vi "Close FPGA Ref.vi"(8 "error in (no error)":errorcluster, 11 "FPGA Ref in":refnum<k20>) -> (0 "error out":errorcluster)   [LabVIEW 2025]
uses:
  <vilib>/FPGAPlugInAG/Dynamic/niLvFpga_Close_Dynamic.vi
  <vilib>/rvi/interface/nirviCloseFPGA/nirviCloseFPGA.xnode
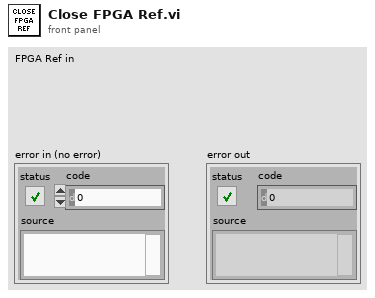
[diagram p1: front panel]
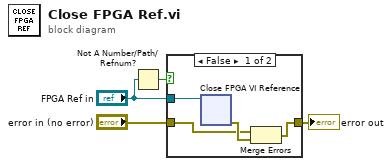
[diagram p0: block diagram]
diagram:
  n1 = Not A Number/Path/Refnum?(number/path/refnum="FPGA Ref in") -> (NaN/Path/Refnum?=w3:bool)
  n2 = case shown="False" w3 {
    tunnel: "FPGA Ref in" -> [w8 _]
    tunnel: "error in (no error)" -> [w5 w9]
    tunnel: [w6 w9] -> w2
    frame False {
      n3 = xnode ("Close FPGA VI Reference")("FPGA VI Reference In"=w8) -> ("error out"=w7:errorcluster)  [unwired: 1 in]
      n4 = Merge Errors(w5, w7) -> (w6:errorcluster)
    }
    frame True {
    }
  }
  "error out" <- w2
